vi "manual head control.vi"() -> ()   [LabVIEW 2017]
panel:
  in  "stop":bool
  in  "Yaw":dbl(slide) scale=-90.0..90.0
  in  "Pitch":dbl(slide) scale=-90.0..90.0
  in  "Roll":dbl(knob) scale=-90.0..90.0
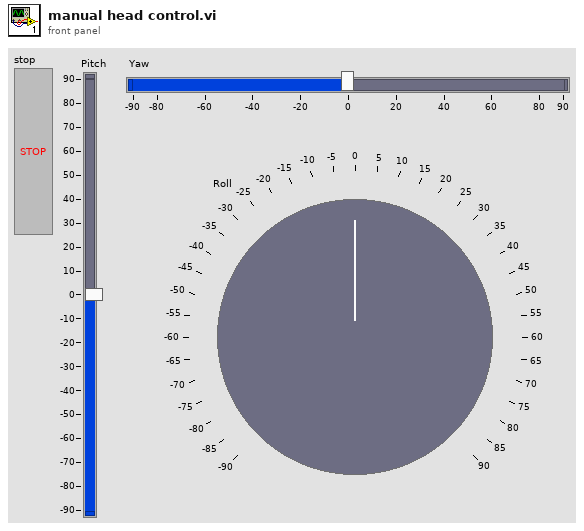
[diagram p1: front panel]
types:
  T1 = cluster{"head":cluster{"orientation":cluster{"roll":dbl, "pitch":dbl, "yaw":dbl}, "position":cluster{"x":dbl, "y":dbl, "z":dbl}}, "hands":cluster{"left":cluster{"position":cluster{"x":dbl, "y":dbl, "z":dbl}, "orientation":cluster{"roll":dbl, "pitch":dbl, "yaw":dbl}}, "right":cluster{"position":cluster{"x":dbl, "y":dbl, "z":dbl}, "orientation":cluster{"roll":dbl, "pitch":dbl, "yaw":dbl}}}, "buttons":cluster{"a":bool, "b":bool, "x":bool, "y":bool, "menu":bool, "leftTrig":dbl, "rightTrig":dbl, "leftGrip":dbl, "rightGrip":dbl, "left_jstick":cluster{"x":dbl, "y":dbl, "button":bool}, "right_jstick":cluster{"x":dbl, "y":dbl, "button":bool}}}
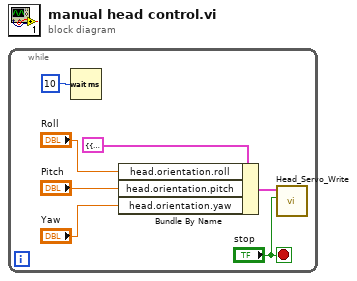
[diagram p0: block diagram]
diagram:
  n1 = while {
    stop <- "stop" stop-if-true
    n2 = Wait (ms)(milliseconds to wait=u32 10) -> ()  [unwired: 1 out]
    n3 = Bundle By Name(cluster=T1 {"head"={"orientation"={"roll"=10.887229431516877, "pitch"=14.275406781509407, "yaw"=-14.676371218055552}, "position"={"x"=0.968743, "y"=0.465524, "z"=-0.764858}}, "hands"={"left"={"position"={"x"=nan, "y"=nan, "z"=nan}, "orientation"={"roll"=11.086045786427272, "pitch"=137.4890151676548, "yaw"=110.57094229039312}}, "right"={"position"={"x"=nan, "y"=nan, "z"=nan}, "orientation"={"roll"=45.66462168036759, "pitch"=106.84098704409148, "yaw"=-80.12597040942414}}}, "buttons"={"a"=FALSE, "b"=FALSE, "x"=FALSE, "y"=FALSE, "menu"=FALSE, "leftTrig"=1e-06, "rightTrig"=1e-06, "leftGrip"=1e-06, "rightGrip"=1e-06, "left_jstick"={"x"=0.0, "y"=0.0, "button"=FALSE}, "right_jstick"={"x"=0.0, "y"=0.0, "button"=FALSE}}} ("Oculus Data in"), "head.orientation.roll"="Roll", "head.orientation.pitch"="Pitch", "head.orientation.yaw"="Yaw") -> (w4:T1)
    n4 = call "Head_Servo_Write.vi"("Stop"="stop", "Calibrated Oculus Data"=w4) -> ()  [unwired: 9 in, 1 out]
  }
